vi "SetLimit_BP4610.vi"(8 "error in":errorcluster, 10 "LimitBP":T1={"Set"=enum."Voltage", "Voltage+[V]"=1.0, "Current+[A]"=-1.0, "Voltage-[V]"=7.0, "Current-[A]"=-7.0} {"Current-[A]" min=-20.0 max=20.0 step=0.001; "Voltage-[V]" min=-115.0 max=115.0 step=0.01; "Current+[A]" min=0.0 max=60.0 step=0.01; "Voltage+[V]" min=0.0 max=120.0 step=0.1}, 11 "VISA":refnum<visa-resource-name> caption="VISAsession") -> (0 "error out":errorcluster, 3 "VISA out":refnum<visa-resource-name>)   [LabVIEW 2019]
uses:
  Type def/limitNF_4610.ctl
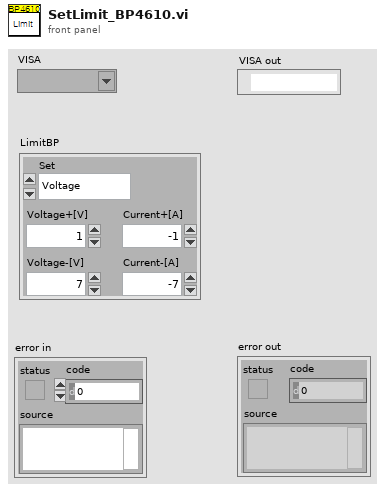
[diagram p1: front panel]
types:
  T1 = typedef "limitNF_4610.ctl" = cluster{"Set":enum16{"Current", "Voltage"}, "Voltage+[V]":dbl, "Current+[A]":dbl, "Voltage-[V]":dbl, "Current-[A]":dbl}
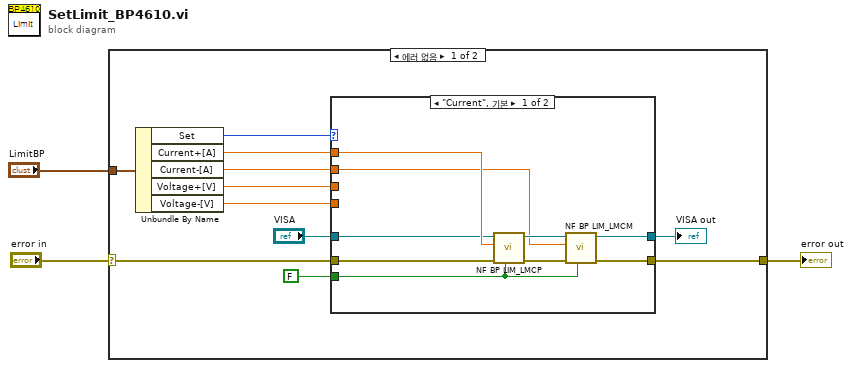
[diagram p0: block diagram]
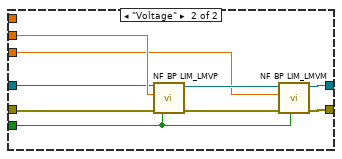
[diagram p2: hidden frame]
diagram:
  n1 = case shown="에러 없음" "error in" {
    selector: "error in" -> [w9 w33]
    tunnel: [w8 w33] -> w2
    tunnel: "LimitBP" -> [w13 _]
    frame No Error {
      n2 = Unbundle By Name(w13) -> ("Set"=w12:enum16{"Current", "Voltage"}, "Current+[A]"=w7:dbl, "Current-[A]"=w6:dbl, "Voltage+[V]"=w11:dbl, "Voltage-[V]"=w10:dbl)
      n3 = case shown="\"Current\", 기본" w12 {
        tunnel: w9 -> [w21 w32]
        tunnel: [w23 w30] -> w8
        tunnel: FALSE ("Read") -> [w20 w29]
        tunnel: [w18 w27] -> w4
        tunnel: w11 -> [_ w26]
        tunnel: w10 -> [_ w25]
        tunnel: w7 -> [w17 _]
        tunnel: w6 -> [w16 _]
        tunnel: "VISA" -> [w15 w24]
        frame "Current", Default {
          n4 = call <instrlib>:"NF BP LIM_LMCP.vi"("Read(F)"=w20, "error in (no error)"=w21, "Current[A]"=w17, "VISAsession"=w15) -> ("error out"=w22:errorcluster, "CopyVISAsession"=w19:refnum<visa-resource-name>)  [unwired: 4 in, 2 out]
          n5 = call <instrlib>:"NF BP LIM_LMCM.vi"("Read(F)"=w20, "error in (no error)"=w22, "Current[A]"=w16, "VISAsession"=w19) -> ("error out"=w23:errorcluster, "CopyVISAsession"=w18:refnum<visa-resource-name>)  [unwired: 4 in, 2 out]
        }
        frame "Voltage" {
          n6 = call <instrlib>:"NF BP LIM_LMVP.vi"("Read(F)"=w29, "error in (no error)"=w32, "Voltage[V]"=w26, "VISAsession"=w24) -> ("error out"=w31:errorcluster, "CopyVISAsession"=w28:refnum<visa-resource-name>)  [unwired: 4 in, 2 out]
          n7 = call <instrlib>:"NF BP LIM_LMVM.vi"("Read(F)"=w29, "error in (no error)"=w31, "Voltage[V]"=w25, "VISAsession"=w28) -> ("error out"=w30:errorcluster, "CopyVISAsession"=w27:refnum<visa-resource-name>)  [unwired: 4 in, 2 out]
        }
      }
      "VISA out" <- w4
    }
    frame Error {
    }
  }
  "error out" <- w2
